vi "normalized PID output.vi"(4 "lower limit":dbl format="%.2f", 5 "upper limit":dbl format="%.2f", 7 "output value":dbl format="%.2f") -> (2 "normalized output value":dbl format="%.2f")   [LabVIEW 2016]
doc: "This subVI normalizes the PID output value from -1 to +1 for the chart."
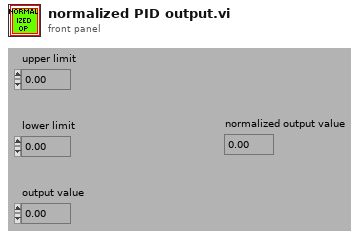
[diagram p1: front panel]
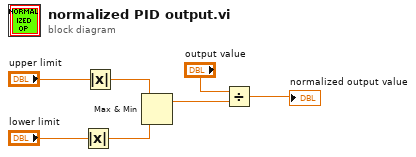
[diagram p0: block diagram]
diagram:
  n1 = Absolute Value(x="lower limit") -> (abs(x)=w4:dbl)
  n2 = Absolute Value(x="upper limit") -> (abs(x)=w3:dbl)
  n3 = Max & Min(x=w3, y=w4) -> (max(x,y)=w5:dbl)  [unwired: 1 out]
  n4 = Divide(x="output value", y=w5) -> (x/y=→"normalized output value":dbl)
